vi "CALCULO FECHAS (SubVI).vi"() -> (1 "años":dbl, 2 "Tiempo actual":timestamp)   [LabVIEW 2018]
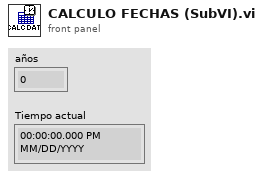
[diagram p1: front panel]
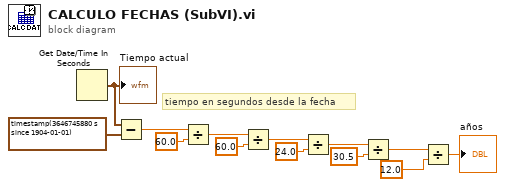
[diagram p0: block diagram]
diagram:
  # "tiempo en segundos desde la fecha"
  n1 = Get Date/Time In Seconds() -> (seconds since 1Jan1904=w1:timestamp)
  "Tiempo actual" <- w1
  n2 = Subtract(x=w1, y=timestamp(3646745880 s since 1904-01-01) ("Tiempo actual 2")) -> (x-y=w3:dbl)
  n3 = Divide(x=w3, y=60.0) -> (x/y=w5:dbl)
  n4 = Divide(x=w5, y=60.0) -> (x/y=w7:dbl)
  n5 = Divide(x=w7, y=24.0) -> (x/y=w9:dbl)
  n6 = Divide(x=w9, y=30.5) -> (x/y=w12:dbl)
  n7 = Divide(x=w12, y=12.0) -> (x/y=→"años":dbl)
